vi "APC_9049_SaveTestAverageValues.vi"(0 "ID":u32, 1 "Data Array":dbl[][](array[numeric])=[[1.0, 0.0, 3.6788, 0.0, 0.0, 0.0, 0.0, 0.0, 0.0, 0.0, 10000000000.0]], 2 "Signals":string[](array[string])=["Cyl1", "", "", "", "", "", "Cyl10"], 3 "PostMortem":bool, 4 "Files and paths":T1, 5 "Test Notes":string="Manual notes along test run.\n\n\n") -> ()   [LabVIEW 2020]
uses:
  <vilib>/Analysis/NI_AALBase.lvlib
panel:
  out "before substring":string
  out "spreadsheet string":string
  out "ERROR 3":bool=TRUE
  out "MAX":dbl[](array[numeric])
  out "MIN":dbl[](array[numeric])
  out "AVG":dbl[](array[numeric])
  out "STD":dbl[](array[numeric])
  out "String to save":string="6\t1.000000\t0.000000\t3.678800\t0.000000\t0.000000\t0.000000\t0.000000\t0.000000\t0.000000\t0.000000\t10000000000.000000\tfile1.tdms\tfile2.tdms\tManual notes along test run._________\r\n"
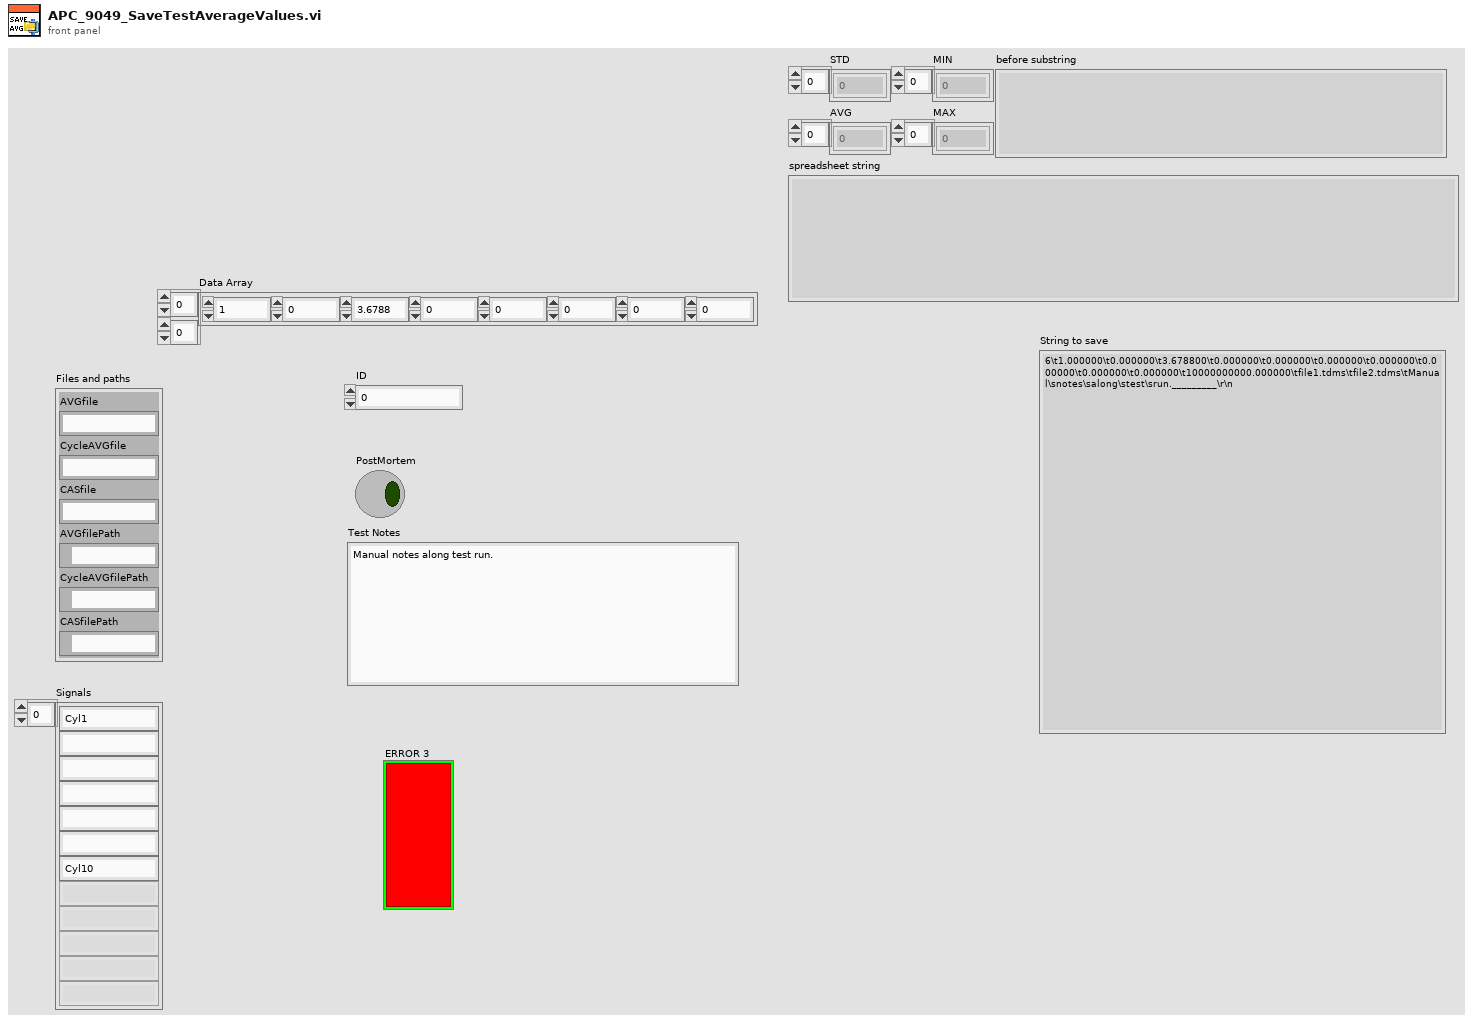
[diagram p1: front panel]
types:
  T1 = cluster{"AVGfile":string, "CycleAVGfile":string, "CASfile":string, "AVGfilePath":path, "CycleAVGfilePath":path, "CASfilePath":path}
  T2 = enum16{"open", "replace", "create", "open or create", "replace or create", "replace or create with confirmation"}
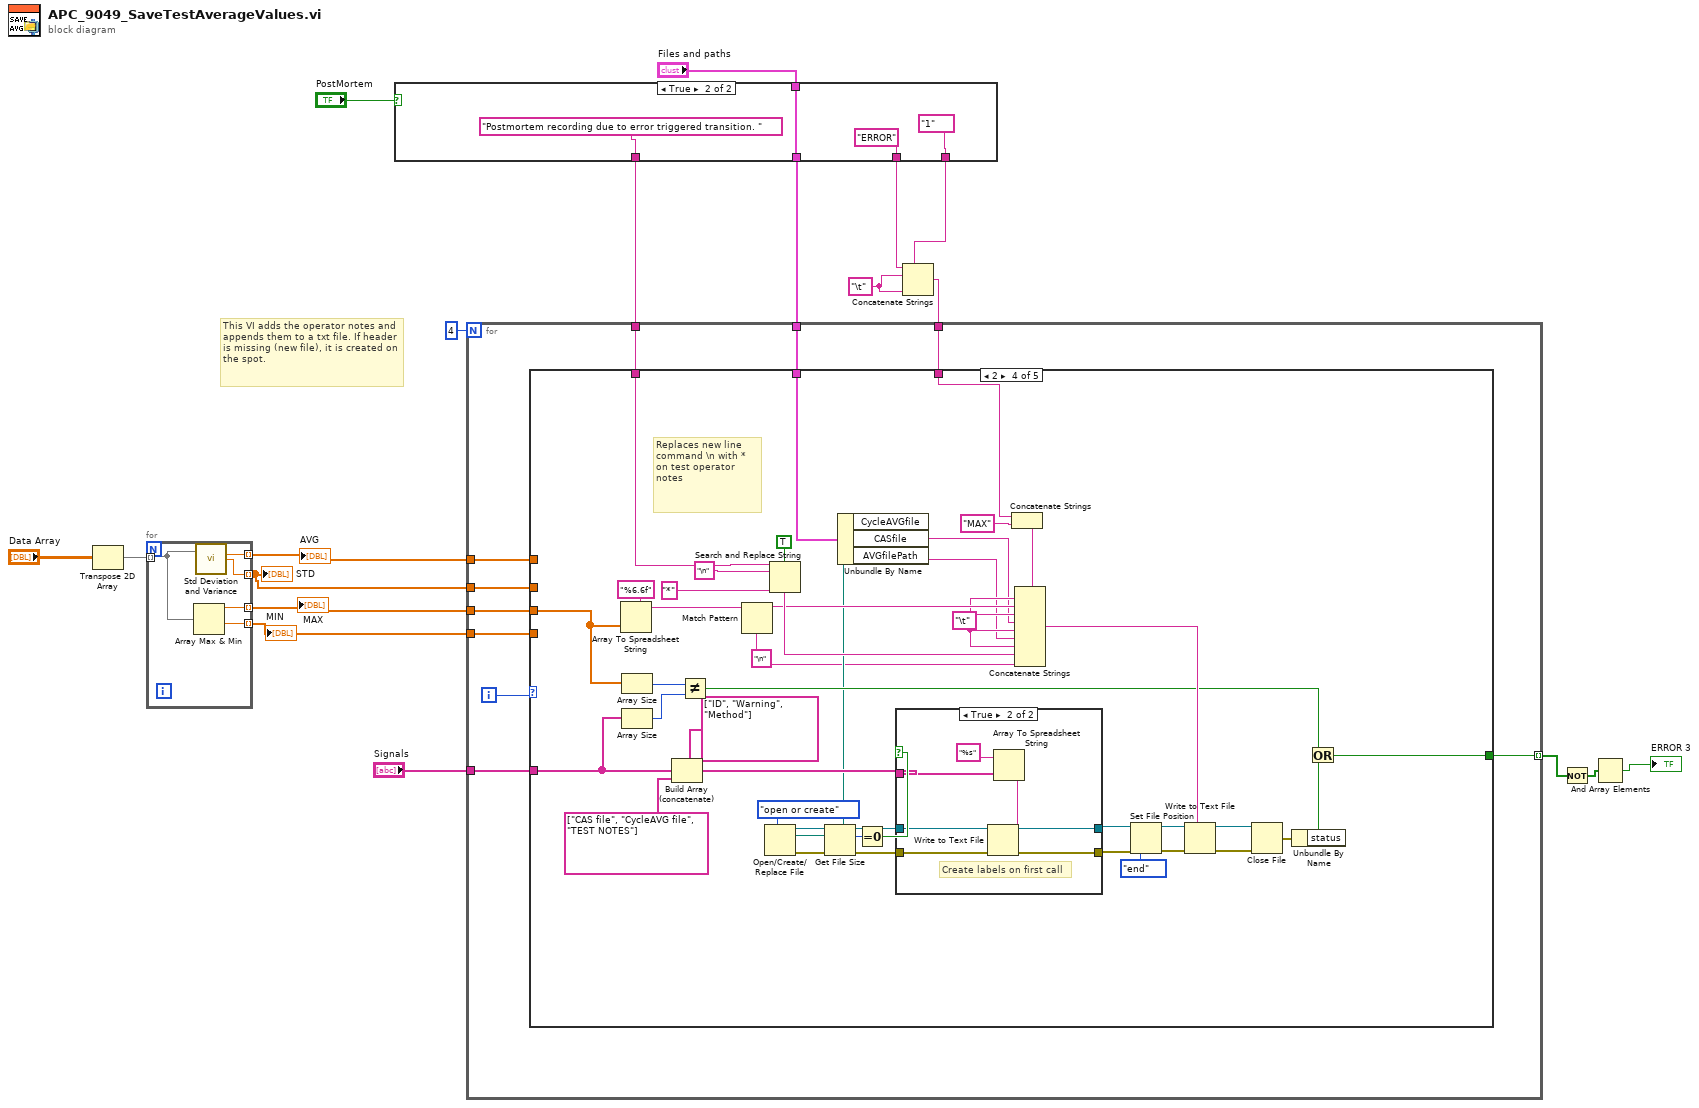
[diagram p0: block diagram]
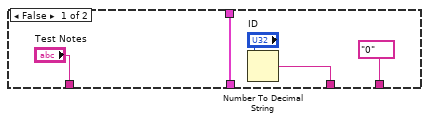
[diagram p2: hidden frame]
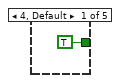
[diagram p3: hidden frame]
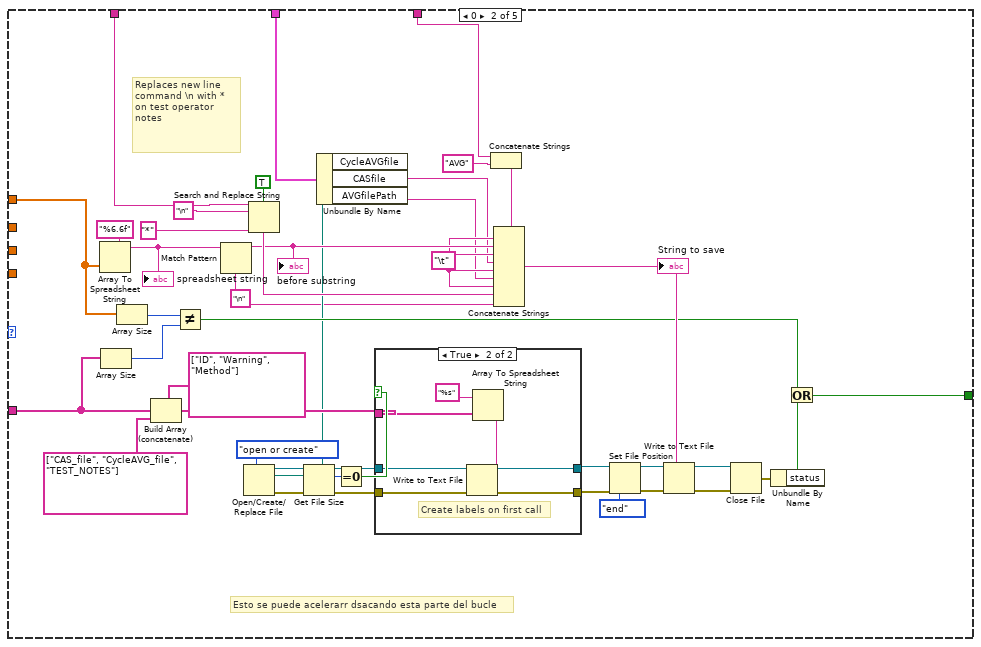
[diagram p4: hidden frame]
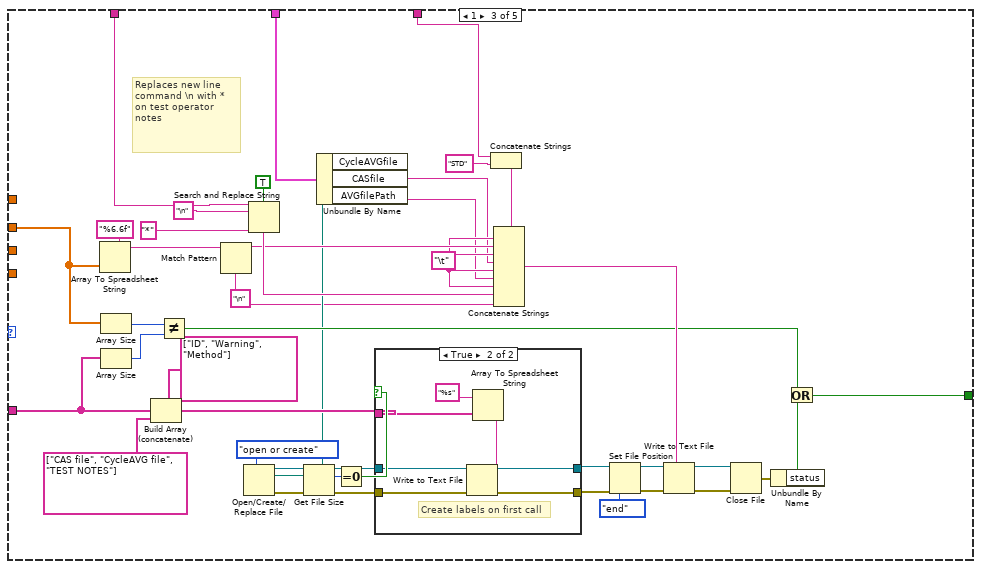
[diagram p6: hidden frame]
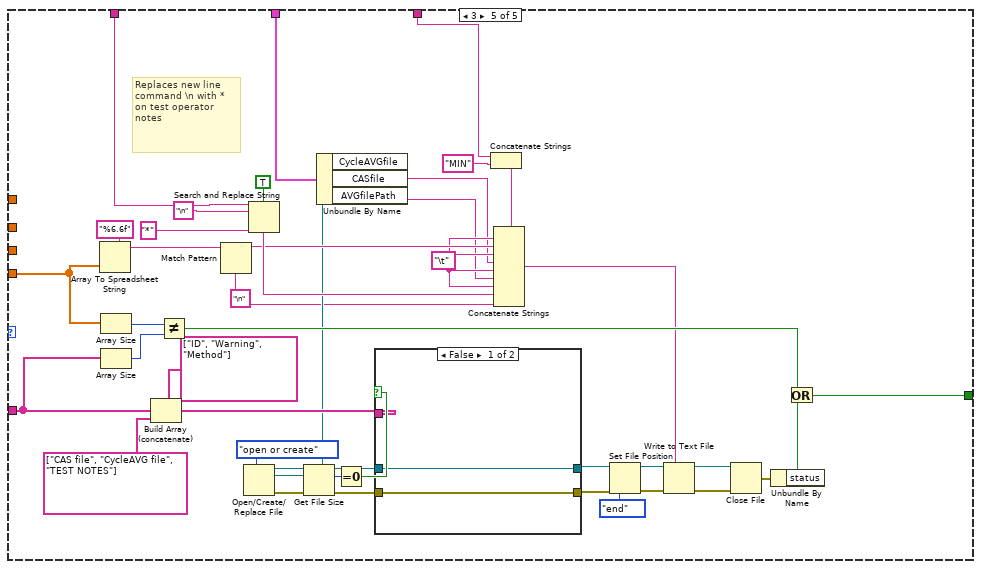
[diagram p9: hidden frame]
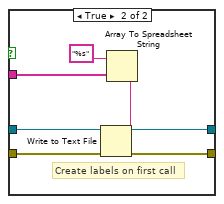
[diagram p10: hidden frame]
diagram:
  w11 = "\t" ("string")
  # "This VI adds the operator notes and appends them to a txt file. If header is missing (new file), it is created on the spot."
  n1 = Transpose 2D Array(2D array="Data Array") -> (transposed array=w17:dbl[][])
  n2 = for {
    tunnel: w17 -> [w22] mode=indexing
    tunnel: [w24] -> w19 mode=indexing
    tunnel: [w23] -> w15 mode=indexing
    tunnel: [w21] -> w14 mode=indexing
    tunnel: [w20] -> w13 mode=indexing
    n3 = Array Max & Min(array=w22) -> (max value=w21:dbl, min value=w20:dbl)  [unwired: 2 out]
    n4 = call <vilib>:"Std Deviation and Variance.vi"("X"=w22) -> ("mean"=w24:dbl, "standard deviation"=w23:dbl)  [unwired: 1 in, 1 out]
  }
  "STD" <- w15
  "AVG" <- w19
  "MIN" <- w13
  "MAX" <- w14
  n5 = case shown="True" "PostMortem" {
    tunnel: ["0" ("decimal integer string") "1" ("decimal integer string")] -> w10
    tunnel: ["Test Notes" "Postmortem recording due to error triggered transition. " ("Test Notes")] -> w4
    tunnel: [w27 w31] -> w3
    tunnel: "Files and paths" -> [w27 w31]
    tunnel: [w25 "ERROR"] -> w1
    frame False {
      n6 = Number To Decimal String(number="ID") -> (decimal integer string=w25:string)  [unwired: 1 in]
    }
    frame True {
    }
  }
  n7 = Concatenate Strings(w1, w11, w10, w11) -> (w9:string)
  n8 = for {
    N: 4 -> [_]
    tunnel: w19 -> [w43]
    tunnel: w15 -> [w40]
    tunnel: w14 -> [w39]
    tunnel: w13 -> [w38]
    tunnel: w3 -> [w42]
    tunnel: w4 -> [w41]
    tunnel: w9 -> [w36]
    tunnel: [w35] -> w8 mode=indexing
    tunnel: "Signals" -> [w34]
    i -> [w37]
    n9 = case shown="2" w37 {
      tunnel: w43 -> [_ w52 _ _ _]
      tunnel: w42 -> [_ w51 w104 w156 w209]
      tunnel: w41 -> [_ w50 w103 w155 w208]
      tunnel: w40 -> [_ _ w100 _ _]
      tunnel: w39 -> [_ _ _ w152 _]
      tunnel: w38 -> [_ _ _ _ w205]
      tunnel: w36 -> [_ w47 w99 w151 w204]
      tunnel: [TRUE w46 w98 w150 w203] -> w35
      tunnel: w34 -> [_ w45 w97 w149 w201]
      frame 4, Default {
      }
      frame 0 {
        w57 = "\t" ("string")
        w53 = "\n" ("regular expression")
        # "Esto se puede acelerarr dsacando esta parte del bucle"
        # "Replaces new line command \\n with *  on test operator notes"
        n10 = Array To Spreadsheet String(array=w52, 3:"%6.6f" ("format string")) -> (spreadsheet string=w85:string)  [unwired: 1 in]
        "spreadsheet string" <- w85
        n11 = Array Size(array=w45) -> (size(s)=w64:i32)
        n12 = Array Size(array=w52) -> (size(s)=w65:i32)
        n13 = Build Array (concatenate)(string[] ["ID", "Warning", "Method"] ("array"), w45, string[] ["CAS_file", "CycleAVG_file", "TEST_NOTES"] ("element")) -> (w67:string[])
        n14 = Not Equal?(x=w65, y=w64) -> (x != y?=w62:bool)
        n15 = Match Pattern(string=w85, regular expression=w53) -> (before substring=w58:string)  [unwired: 1 in, 3 out]
        "before substring" <- w58
        n16 = Search and Replace String(replace all?=TRUE ("replace all? (F)"), input string=w50, search string="\n", replace string="*" ("replace string (\"\")")) -> (result string=w77:string)  [unwired: 4 in, 3 out]
        n17 = Unbundle By Name(w51) -> ("CycleAVGfile"=w56:string, "CASfile"=w55:string, "AVGfilePath"=w54:path)
        n18 = Open/Create/Replace File(file path (use dialog)=w54, operation (0:open)=T2."open or create") -> (refnum out=w78:refnum<file>, error out=w61:errorcluster)  [unwired: 4 in, 1 out]
        n19 = Get File Size(file=w78, error in=w61) -> (refnum out=w72:refnum<file>, size (in bytes)=w74:i64, 0:w71:errorcluster)
        n20 = Equal To 0?(x=w74) -> (x = 0?=w73:bool)
        n21 = case shown="True" w73 {
          tunnel: w72 -> [w89 w96]
          tunnel: w71 -> [w88 w95]
          tunnel: [w89 w94] -> w70
          tunnel: [w88 w93] -> w69
          tunnel: w67 -> [_ w92]
          frame False {
          }
          frame True {
            # "Create labels on first call"
            n22 = Array To Spreadsheet String(array=w92, 3:"%s" ("format string")) -> (spreadsheet string=w91:string)  [unwired: 1 in]
            n23 = Write to Text File(file (use dialog)=w96, text=w91, error in=w95) -> (refnum out=w94:refnum<file>, error out=w93:errorcluster)  [unwired: 1 in, 1 out]
          }
        }
        n24 = Concatenate Strings(w47, "AVG" ("string")) -> (w48:string)
        n25 = Concatenate Strings(w48, w57, w58, w57, w55, w57, w56, w57, w77, w53) -> (w86:string)
        "String to save" <- w86
        n26 = Set File Position(refnum=w70, from (0:start)=enum16{"start", "end", "current"}."end", error in=w69) -> (refnum out=w82:refnum<file>, error out=w81:errorcluster)  [unwired: 1 in]
        n27 = Write to Text File(file (use dialog)=w82, text=w86, error in=w81) -> (refnum out=w80:refnum<file>, error out=w79:errorcluster)  [unwired: 1 in, 1 out]
        n28 = Close File(refnum=w80, error in=w79) -> (error out=w66:errorcluster)  [unwired: 1 out]
        n29 = Unbundle By Name(w66) -> ("status"=w63:bool)
        n30 = Or(x=w62, y=w63) -> (x .or. y?=w46:bool)
      }
      frame 1 {
        w109 = "\t" ("string")
        w105 = "\n" ("regular expression")
        # "Replaces new line command \\n with *  on test operator notes"
        n31 = Array To Spreadsheet String(array=w100, 3:"%6.6f" ("format string")) -> (spreadsheet string=w137:string)  [unwired: 1 in]
        n32 = Array Size(array=w100) -> (size(s)=w117:i32)
        n33 = Array Size(array=w97) -> (size(s)=w116:i32)
        n34 = Build Array (concatenate)(string[] ["ID", "Warning", "Method"] ("array"), w97, string[] ["CAS file", "CycleAVG file", "TEST NOTES"] ("element")) -> (w119:string[])
        n35 = Not Equal?(x=w117, y=w116) -> (x != y?=w114:bool)
        n36 = Match Pattern(string=w137, regular expression=w105) -> (before substring=w110:string)  [unwired: 1 in, 3 out]
        n37 = Search and Replace String(replace all?=TRUE ("replace all? (F)"), input string=w103, search string="\n", replace string="*" ("replace string (\"\")")) -> (result string=w129:string)  [unwired: 4 in, 3 out]
        n38 = Unbundle By Name(w104) -> ("CycleAVGfile"=w108:string, "CASfile"=w107:string, "AVGfilePath"=w106:path)
        n39 = Open/Create/Replace File(file path (use dialog)=w106, operation (0:open)=T2."open or create") -> (refnum out=w130:refnum<file>, error out=w113:errorcluster)  [unwired: 4 in, 1 out]
        n40 = Get File Size(file=w130, error in=w113) -> (refnum out=w124:refnum<file>, size (in bytes)=w126:i64, 0:w123:errorcluster)
        n41 = Equal To 0?(x=w126) -> (x = 0?=w125:bool)
        n42 = case shown="True" w125 {
          tunnel: w124 -> [w141 w148]
          tunnel: w123 -> [w140 w147]
          tunnel: [w141 w146] -> w122
          tunnel: [w140 w145] -> w121
          tunnel: w119 -> [_ w144]
          frame False {
          }
          frame True {
            # "Create labels on first call"
            n43 = Array To Spreadsheet String(array=w144, 3:"%s" ("format string")) -> (spreadsheet string=w143:string)  [unwired: 1 in]
            n44 = Write to Text File(file (use dialog)=w148, text=w143, error in=w147) -> (refnum out=w146:refnum<file>, error out=w145:errorcluster)  [unwired: 1 in, 1 out]
          }
        }
        n45 = Concatenate Strings(w99, "STD" ("string")) -> (w101:string)
        n46 = Concatenate Strings(w101, w109, w110, w109, w107, w109, w108, w109, w129, w105) -> (w138:string)
        n47 = Set File Position(refnum=w122, from (0:start)=enum16{"start", "end", "current"}."end", error in=w121) -> (refnum out=w134:refnum<file>, error out=w133:errorcluster)  [unwired: 1 in]
        n48 = Write to Text File(file (use dialog)=w134, text=w138, error in=w133) -> (refnum out=w132:refnum<file>, error out=w131:errorcluster)  [unwired: 1 in, 1 out]
        n49 = Close File(refnum=w132, error in=w131) -> (error out=w118:errorcluster)  [unwired: 1 out]
        n50 = Unbundle By Name(w118) -> ("status"=w115:bool)
        n51 = Or(x=w114, y=w115) -> (x .or. y?=w98:bool)
      }
      frame 2 {
        w161 = "\t" ("string")
        w157 = "\n" ("regular expression")
        # "Replaces new line command \\n with *  on test operator notes"
        n52 = Array To Spreadsheet String(array=w152, 3:"%6.6f" ("format string")) -> (spreadsheet string=w189:string)  [unwired: 1 in]
        n53 = Array Size(array=w152) -> (size(s)=w169:i32)
        n54 = Array Size(array=w149) -> (size(s)=w168:i32)
        n55 = Build Array (concatenate)(string[] ["ID", "Warning", "Method"] ("array"), w149, string[] ["CAS file", "CycleAVG file", "TEST NOTES"] ("element")) -> (w171:string[])
        n56 = Not Equal?(x=w169, y=w168) -> (x != y?=w166:bool)
        n57 = Match Pattern(string=w189, regular expression=w157) -> (before substring=w162:string)  [unwired: 1 in, 3 out]
        n58 = Search and Replace String(replace all?=TRUE ("replace all? (F)"), input string=w155, search string="\n", replace string="*" ("replace string (\"\")")) -> (result string=w181:string)  [unwired: 4 in, 3 out]
        n59 = Unbundle By Name(w156) -> ("CycleAVGfile"=w160:string, "CASfile"=w159:string, "AVGfilePath"=w158:path)
        n60 = Open/Create/Replace File(file path (use dialog)=w158, operation (0:open)=T2."open or create") -> (refnum out=w182:refnum<file>, error out=w165:errorcluster)  [unwired: 4 in, 1 out]
        n61 = Get File Size(file=w182, error in=w165) -> (refnum out=w176:refnum<file>, size (in bytes)=w178:i64, 0:w175:errorcluster)
        n62 = Equal To 0?(x=w178) -> (x = 0?=w177:bool)
        n63 = case shown="True" w177 {
          tunnel: w176 -> [w193 w200]
          tunnel: w175 -> [w192 w199]
          tunnel: [w193 w198] -> w174
          tunnel: [w192 w197] -> w173
          tunnel: w171 -> [_ w196]
          frame False {
          }
          frame True {
            # "Create labels on first call"
            n64 = Array To Spreadsheet String(array=w196, 3:"%s" ("format string")) -> (spreadsheet string=w195:string)  [unwired: 1 in]
            n65 = Write to Text File(file (use dialog)=w200, text=w195, error in=w199) -> (refnum out=w198:refnum<file>, error out=w197:errorcluster)  [unwired: 1 in, 1 out]
          }
        }
        n66 = Concatenate Strings(w151, "MAX" ("string")) -> (w153:string)
        n67 = Concatenate Strings(w153, w161, w162, w161, w159, w161, w160, w161, w181, w157) -> (w190:string)
        n68 = Set File Position(refnum=w174, from (0:start)=enum16{"start", "end", "current"}."end", error in=w173) -> (refnum out=w186:refnum<file>, error out=w185:errorcluster)  [unwired: 1 in]
        n69 = Write to Text File(file (use dialog)=w186, text=w190, error in=w185) -> (refnum out=w184:refnum<file>, error out=w183:errorcluster)  [unwired: 1 in, 1 out]
        n70 = Close File(refnum=w184, error in=w183) -> (error out=w170:errorcluster)  [unwired: 1 out]
        n71 = Unbundle By Name(w170) -> ("status"=w167:bool)
        n72 = Or(x=w166, y=w167) -> (x .or. y?=w150:bool)
      }
      frame 3 {
        w214 = "\t" ("string")
        w210 = "\n" ("regular expression")
        # "Replaces new line command \\n with *  on test operator notes"
        n73 = Array To Spreadsheet String(array=w205, 3:"%6.6f" ("format string")) -> (spreadsheet string=w242:string)  [unwired: 1 in]
        n74 = Array Size(array=w205) -> (size(s)=w222:i32)
        n75 = Array Size(array=w201) -> (size(s)=w221:i32)
        n76 = Build Array (concatenate)(string[] ["ID", "Warning", "Method"] ("array"), w201, string[] ["CAS file", "CycleAVG file", "TEST NOTES"] ("element")) -> (w224:string[])
        n77 = Not Equal?(x=w222, y=w221) -> (x != y?=w219:bool)
        n78 = Match Pattern(string=w242, regular expression=w210) -> (before substring=w215:string)  [unwired: 1 in, 3 out]
        n79 = Search and Replace String(replace all?=TRUE ("replace all? (F)"), input string=w208, search string="\n", replace string="*" ("replace string (\"\")")) -> (result string=w234:string)  [unwired: 4 in, 3 out]
        n80 = Unbundle By Name(w209) -> ("CycleAVGfile"=w213:string, "CASfile"=w212:string, "AVGfilePath"=w211:path)
        n81 = Open/Create/Replace File(file path (use dialog)=w211, operation (0:open)=T2."open or create") -> (refnum out=w235:refnum<file>, error out=w218:errorcluster)  [unwired: 4 in, 1 out]
        n82 = Get File Size(file=w235, error in=w218) -> (refnum out=w229:refnum<file>, size (in bytes)=w231:i64, 0:w228:errorcluster)
        n83 = Equal To 0?(x=w231) -> (x = 0?=w230:bool)
        n84 = case shown="False" w230 {
          tunnel: w229 -> [w245 w252]
          tunnel: w228 -> [w244 w251]
          tunnel: [w245 w250] -> w227
          tunnel: [w244 w249] -> w226
          tunnel: w224 -> [_ w248]
          frame False {
          }
          frame True {
            # "Create labels on first call"
            n85 = Array To Spreadsheet String(array=w248, 3:"%s" ("format string")) -> (spreadsheet string=w247:string)  [unwired: 1 in]
            n86 = Write to Text File(file (use dialog)=w252, text=w247, error in=w251) -> (refnum out=w250:refnum<file>, error out=w249:errorcluster)  [unwired: 1 in, 1 out]
          }
        }
        n87 = Concatenate Strings(w204, "MIN" ("string")) -> (w206:string)
        n88 = Concatenate Strings(w206, w214, w215, w214, w212, w214, w213, w214, w234, w210) -> (w202:string)
        n89 = Set File Position(refnum=w227, from (0:start)=enum16{"start", "end", "current"}."end", error in=w226) -> (refnum out=w239:refnum<file>, error out=w238:errorcluster)  [unwired: 1 in]
        n90 = Write to Text File(file (use dialog)=w239, text=w202, error in=w238) -> (refnum out=w237:refnum<file>, error out=w236:errorcluster)  [unwired: 1 in, 1 out]
        n91 = Close File(refnum=w237, error in=w236) -> (error out=w223:errorcluster)  [unwired: 1 out]
        n92 = Unbundle By Name(w223) -> ("status"=w220:bool)
        n93 = Or(x=w219, y=w220) -> (x .or. y?=w203:bool)
      }
    }
  }
  n94 = Not(x=w8) -> (.not. x?=w7:bool[])
  n95 = And Array Elements(Boolean array=w7) -> (logical AND=→"ERROR 3":bool)
